vi "fill in mising device data.vi"(9 "shot #s main":string[](array[string]), 10 "total # shots":i32, 11 "devive data in":string[][](array[string])) -> (3 "Array":string[][](array[string]))   [LabVIEW 2018]
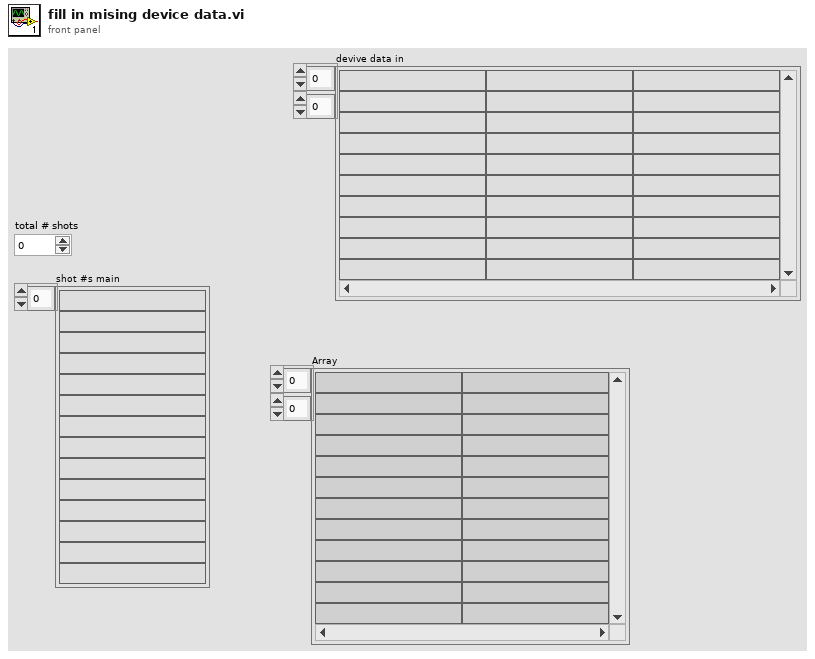
[diagram p1: front panel]
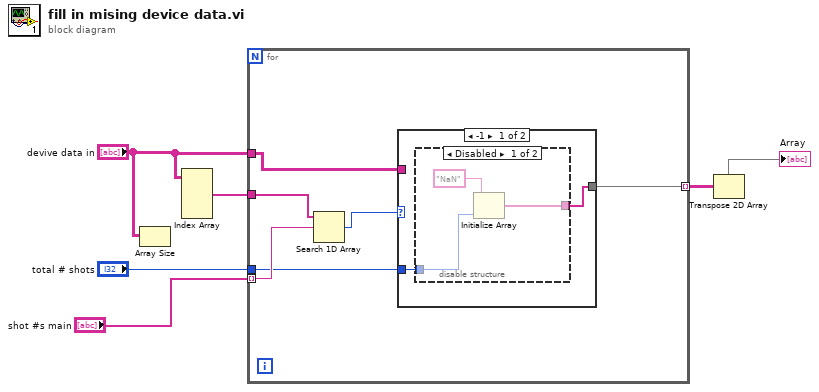
[diagram p0: block diagram]
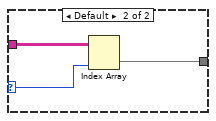
[diagram p3: hidden frame]
diagram:
  n1 = Array Size(array="devive data in") -> ()  [unwired: 1 out]
  n2 = Index Array(array="devive data in") -> (element #1=w3:string[])  [unwired: 4 in, 1 out]
  n3 = for {
    tunnel: "shot #s main" -> [w11] mode=indexing
    tunnel: "devive data in" -> [w10]
    tunnel: w3 -> [w12]
    tunnel: [w8] -> w4 mode=indexing
    tunnel: "total # shots" -> [w7]
    n4 = Search 1D Array(1D array=w12, element=w11) -> (index of element=w9:i32)  [unwired: 1 in]
    n5 = case shown="-1" w9 {
      selector: w9 -> [_ w19]
      tunnel: w10 -> [_ w20]
      tunnel: [w13 w18] -> w8
      tunnel: w7 -> [w14 _]
      frame -1 {
        n6 = disable-structure shown="Disabled" {
          disable-tunnel: w14 -> [w16 _]
          disable-tunnel: [w15 _] -> w13
          frame Disabled {
            n7 = Initialize Array("NaN", w16) -> (w15:string[])
          }
          frame Enabled {
          }
        }
      }
      frame Default {
        n8 = Index Array(array=w20, index (col)=w19) -> (element=w18:string[])  [unwired: 1 in]
      }
    }
  }
  n9 = Transpose 2D Array(2D array=w4) -> (transposed array=→"Array":string[][])
